vi "Delete All Display Objects.vi"(8 "Error In":errorcluster, 11 "Display Manager In":refnum<class "Display Manager.lvclass">) -> (0 "Error Out":errorcluster, 3 "Display Manager Out":refnum<class "Display Manager.lvclass">)   [LabVIEW 2021, in "Display Manager.lvclass"]
uses:
  Display Manager.lvclass
  Accessors/Display/Get Display.vi
  <vilib>/Memosfet/myRIO-Neopixel/RT/Display/Display.lvclass
  <vilib>/Memosfet/myRIO-Neopixel/RT/Display Element/Display Element.lvclass
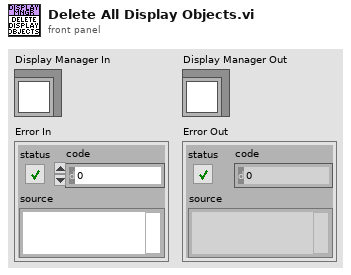
[diagram p1: front panel]
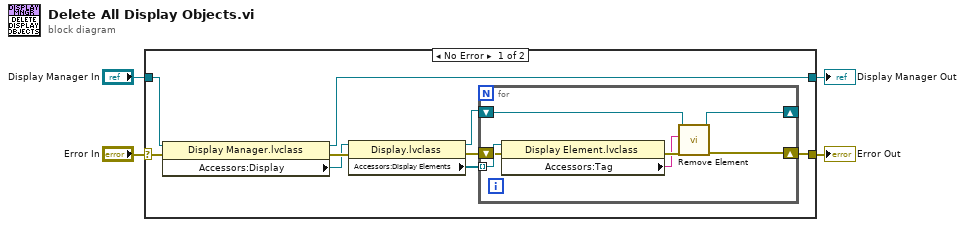
[diagram p0: block diagram]
diagram:
  n1 = case shown="No Error" "Error In" {
    selector: "Error In" -> [w12 w22]
    tunnel: [w5 w22] -> w3
    tunnel: "Display Manager In" -> [w13 w21]
    tunnel: [w11 w21] -> w1
    frame No Error {
      n2 = property class="Display Manager.lvclass"(reference=w13, error in=w12) -> (reference out=w11:refnum<class "Display Manager.lvclass">, error out=w10:errorcluster, "Accessors:Display"=w9:refnum<class "Display.lvclass">)
      n3 = property class="Display.lvclass"(reference=w9, error in=w10) -> (reference out=w6:refnum<class "Display.lvclass">, error out=w7:errorcluster, "Accessors:Display Elements"=w8:refnum<class "Display Element.lvclass">[])
      n4 = for {
        tunnel: w8 -> [w20] mode=indexing
        shift-right: [w14] -> w5
        shift-left: w7 -> [w19]
        shift-right: [w17] -> _
        shift-left: w6 -> [w18]
        n5 = property class="Display Element.lvclass"(reference=w20, error in=w19) -> (error out=w16:errorcluster, "Accessors:Tag"=w15:string)  [unwired: 1 out]
        n6 = call <vilib>:"Remove Element.vi"("Error In"=w16, "Element Tag"=w15, "Display In"=w18) -> ("Error Out"=w14:errorcluster, "Display Out"=w17:refnum<class "Display.lvclass">)  [unwired: 7 in]
      }
    }
    frame Error {
    }
  }
  "Display Manager Out" <- w1
  "Error Out" <- w3
